vi "test_v2.vi"() -> ()   [LabVIEW 2025]
uses:
  <vilib>/Instr/_visa.llb/VISA Configure Serial Port (Instr).vi
panel:
  out "read buffer":string
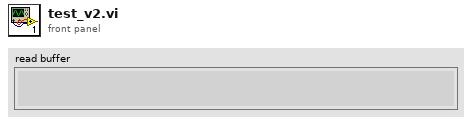
[diagram p1: front panel]
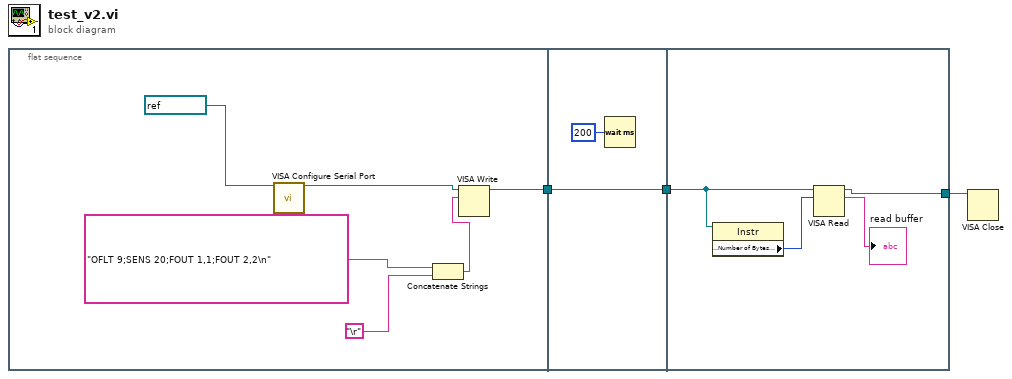
[diagram p0: block diagram]
diagram:
  n1 = flat-sequence {
    tunnel: [w4] -> w3
    tunnel: w3 -> [w11]
    tunnel: [w11] -> w2
    tunnel: w2 -> [w14]
    tunnel: [w13] -> w1
    frame #0 {
      n2 = call-poly "VISA Configure Serial Port"("VISA resource name"=refnum<visa-resource-name> "COM1") -> ("VISA resource name out"=w8:refnum<visa-resource-name>)  [unwired: 13 in, 1 out]
      n3 = Concatenate Strings("OFLT 9;SENS 20;FOUT 1,1;FOUT 2,2\n" ("write buffer"), "\r") -> (w5:string)
      n4 = VISA Write(VISA resource name=w8, write buffer=w5) -> (VISA resource name out=w4:refnum<visa-resource-name>)  [unwired: 1 in, 2 out]
    }
    frame #1 {
      n5 = Wait (ms)(milliseconds to wait=u32 200) -> ()  [unwired: 1 out]
    }
    frame #2 {
      n6 = property class="Instr"(reference=w14) -> ("Serial Settings:Number of Bytes at Serial Port"=w15:u32)  [unwired: 1 in, 2 out]
      n7 = VISA Read(VISA resource name=w14, byte count=w15) -> (VISA resource name out=w13:refnum<visa-resource-name>, read buffer=→"read buffer":string)  [unwired: 1 in, 2 out]
    }
  }
  n8 = VISA Close(VISA resource name=w1) -> ()  [unwired: 1 in, 1 out]
